vi "NMR T2 CPMG Sequence - Large Magnet - MC HPA (2W) - 2nd Setup.vi"() -> ()   [LabVIEW 2020]
uses:
  <instrlib>/niFgen/niFgen.llb/niFgen Output Mode.ctl
  <instrlib>/niFgen/niFgen.llb/niFgen Waveform Type.ctl
  <instrlib>/niFgen/niFgen.llb/niFgen_ctl Trigger DigEdge - Edge Values (Ring).ctl
  <instrlib>/niFgen/niFgen.llb/niFgen_ctl Trigger Source Values (Ring).ctl
  <instrlib>/niFgen/niFgen.llb/niFgen Trigger Mode.ctl
  <instrlib>/niScope/Controls/niScope acquisition type.ctl
  <instrlib>/niScope/Controls/niScope trigger slope.ctl
  <instrlib>/niScope/Controls/niScope trigger source.ctl
  <vilib>/Analysis/2dsp.llb/Integral Method.ctl
  <vilib>/Analysis/8numeric.llb/1D Numeric Integration.vi
  <vilib>/Utility/file.llb/Read Delimited Spreadsheet (DBL).vi
  <instrlib>/niFgen/niFgen.llb/niFgen Create Waveform (DBL).vi
  <instrlib>/niScope/Configure/Trigger/niScope Configure Trigger Edge.vi
  <instrlib>/niFgen/niFgen.llb/niFgen Configure Digital Edge Start Trigger.vi
  <instrlib>/niScope/Acquire/Fetch/niScope Fetch Cluster.vi
  <vilib>/Waveform/WDTFileIO.llb/Export Waveform To Spreadsheet File.vi
  <vilib>/Analysis/NI_AALPro.lvlib
panel:
  out "Pulse Echos - Current Scan":waveform(dbl)(graph)={"t0"=timestamp(0 s since 1904-01-01), "dt"=0.0012610340479192938, "Y"=array[3965 elements]} caption="Waveform Graph"
  in  "Write Output to File?":bool=TRUE
  out "Averaged T2 Decay":waveform(dbl)(graph)={"t0"=timestamp(0 s since 1904-01-01), "dt"=0.0012610340479192938, "Y"=array[3965 elements]} caption="Waveform Graph"
  out "Scan Number":i32=8
  out "Signal Intensity (Integral)":dbl=0.6544283602926818 format="%0.4f"
  out "Extracted T2 Decay - Current Scan":waveform(dbl)(graph)={"t0"=timestamp(0 s since 1904-01-01), "dt"=0.0012610340479192938, "Y"=array[3965 elements]} caption="Waveform Graph"
  in  "Pulse Train File":path=path "C:/Users/localuser/OneDrive - University of South Carolina/NMR Research/MATLAB/6 us 90 Degree - 1.25ms Tau - 3965 Pulses.txt"
  in  "Larmor Frequency":dbl=27410000.0 caption="Frequency" format="%.4p"
  in  "Number of Scans":i32=8
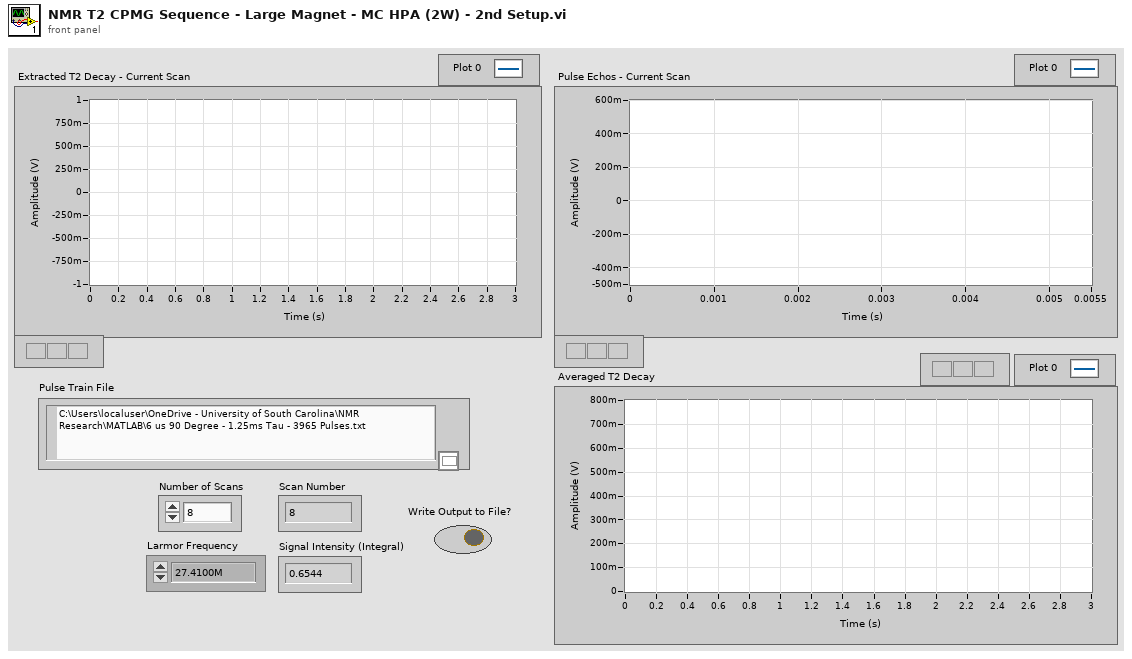
[diagram p1: front panel]
types:
  T1 = typedef "niFgen Output Mode.ctl" = u32
  T2 = typedef "niScope trigger source.ctl" = string
  T3 = typedef "niFgen_ctl Trigger Source Values (Ring).ctl" = string
  T4 = typedef "NI_AALPro.lvlib/Integral Method.ctl" = i32
  T5 = typedef "niScope trigger slope.ctl" = i32
  T6 = typedef "niScope acquisition type.ctl" = i32
  T7 = typedef "niFgen Trigger Mode.ctl" = i32
  T8 = typedef "niFgen_ctl Trigger DigEdge - Edge Values (Ring).ctl" = i32
  T9 = typedef "niFgen Waveform Type.ctl" = i32
  T10 = cluster{"relativeInitialX":dbl, "xIncrement":dbl, "wfm":dbl[]}
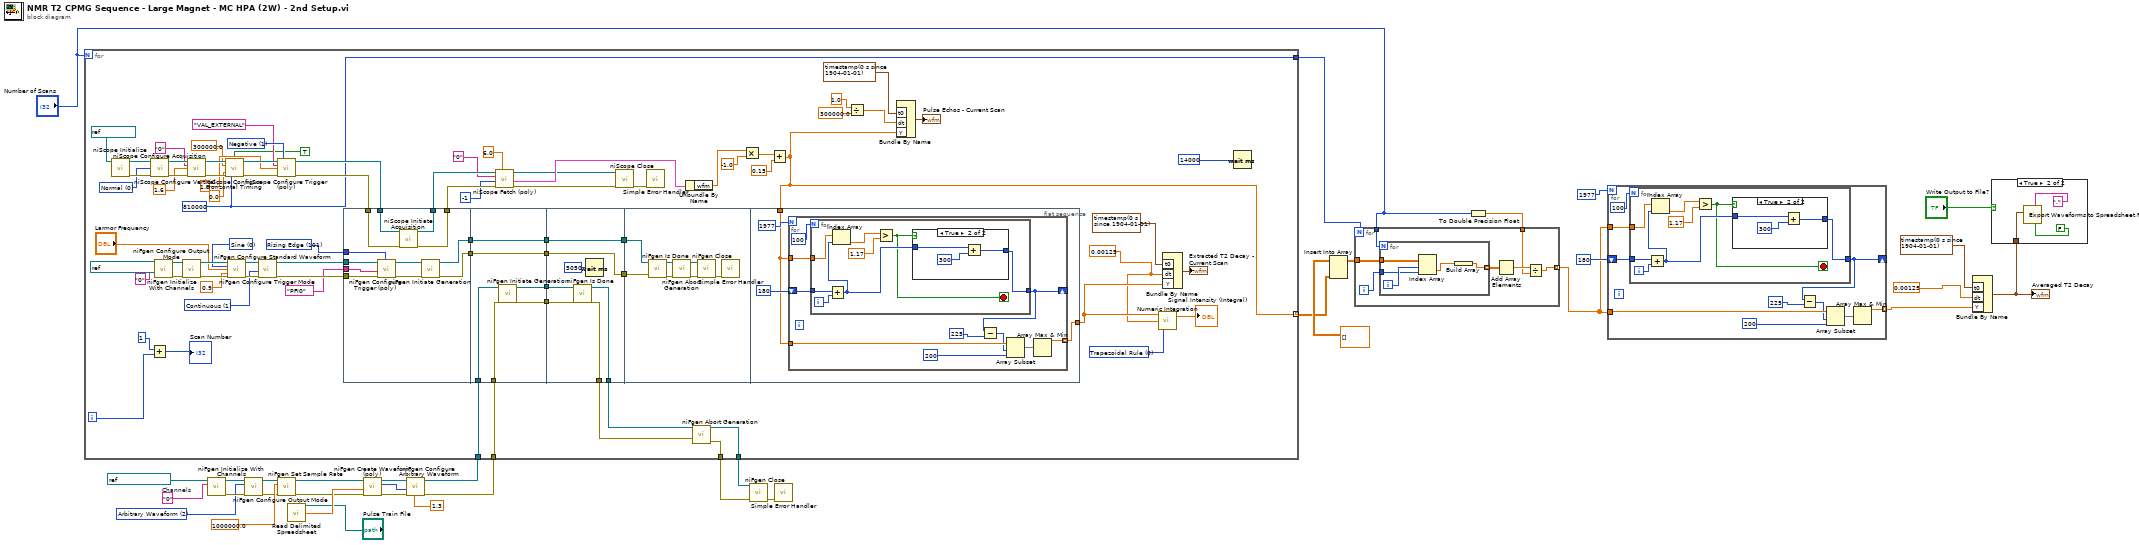
[diagram p0: block diagram]
diagram:
  w21 = "0"  # Channels
  w20 = T1 2 items=["Standard Function", "Frequency List", "Arbitrary Waveform", "Arbitrary Sequence", "Script"] ("output mode")
  n1 = call <instrlib>:"niFgen Initialize With Channels.vi"("Channel Name"=w21, "Resource Name"=refnum<k15> "PulseGenerator" ("FGEN Resource Name 2")) -> ("error out"=w24:errorcluster, "Instrument Handle Out"=w25:refnum<k15>)  [unwired: 8 in]
  n2 = call <instrlib>:"niFgen Configure Output Mode.vi"("error in (no error)"=w24, "Output Mode (default: 0=Standard Function)"=w20, "Instrument Handle"=w25) -> ("error out"=w28:errorcluster, "Instrument Handle Out"=w27:refnum<k15>)  [unwired: 6 in]
  n3 = call <instrlib>:"niFgen Set Sample Rate.vi"("error in (no error)"=w28, "Sample Rate (Samp/s)"=1000000.0 ("Sample Rate"), "Instrument Handle"=w27) -> ("error out"=w31:errorcluster, "Instrument Handle Out"=w30:refnum<k15>)  [unwired: 7 in]
  n4 = call-poly <vilib>:"Read Delimited Spreadsheet.vi"("file path (dialog if empty)"="Pulse Train File") -> ("first row"=w32:dbl[])  [unwired: 9 in, 5 out]
  n5 = call-poly <instrlib>:"niFgen Create Waveform (poly).vi"("error in (no error)"=w31, "Waveform Data Array"=w32, "Instrument Handle"=w30) -> ("error out"=w34:errorcluster, "Waveform Handle"=w35:i32, "Instrument Handle Out"=w33:refnum<k15>)  [unwired: 6 in]
  n6 = call <instrlib>:"niFgen Configure Arbitrary Waveform.vi"("Gain"=1.3, "error in (no error)"=w34, "Waveform Handle"=w35, "Instrument Handle"=w33) -> ("error out"=w19:errorcluster, "Instrument Handle Out"=w18:refnum<k15>)  [unwired: 6 in]
  n7 = for {
    N: "Number of Scans" -> [_]
    tunnel: w19 -> [w97]
    tunnel: w18 -> [w96]
    tunnel: [w95] -> w16
    tunnel: [w94] -> w15
    tunnel: [w37] -> w12 mode=indexing
    tunnel: [w48] -> w9
    i -> [w55]
    w57 = T4 0 items=["Trapezoidal Rule", "Simpson's Rule", "Simpson's 3/8 Rule", "Bode Rule"] ("integration method")
    w36 = 0.00125 ("y")
    w48 = 810000 ("min record length")
    w82 = T5 1 items=["Positive", "Negative"] ("trigger slope")
    w83 = T6 0 items=["Normal"=0, "Flex Res"=1, "DDC"=3] ("acquisition Type")
    w102 = T7 1 items=["Single", "Continuous", "Stepped", "Burst"] ("Trigger Mode (default: 1=continuous)")
    w106 = T8 101 items=["Rising Edge"=101, "Falling Edge"=102] ("Edge (Rising)")
    w107 = T9 0 items=["Sine", "Square", "Triangle", "Ramp Up", "Ramp Down", "DC", "Noise", "User"] ("Waveform")
    n8 = call <instrlib>:"niScope Initialize.vi"("resource name"=refnum<k15> "PXI1Slot6") -> ("instrument handle"=w84:refnum<k15>, "error out"=w85:errorcluster)  [unwired: 13 in]
    n9 = call <instrlib>:"niScope Configure Acquisition.vi"("instrument handle"=w84, "acquisition Type"=w83, "error in"=w85) -> ("instrument handle out"=w87:refnum<k15>, "error out"=w88:errorcluster)  [unwired: 11 in]
    n10 = Add(x=1, y=w55) -> (x+y=→"Scan Number":i32)
    n11 = call <instrlib>:"niFgen Initialize With Channels.vi"("Channel Name"="0", "Resource Name"=refnum<k15> "SinWaveGenerator" ("Sine Wave Module")) -> ("error out"=w112:errorcluster, "Instrument Handle Out"=w115:refnum<k15>)  [unwired: 8 in]
    n12 = call <instrlib>:"niFgen Configure Output Mode.vi"("error in (no error)"=w112, "Instrument Handle"=w115) -> ("error out"=w111:errorcluster, "Instrument Handle Out"=w114:refnum<k15>)  [unwired: 7 in]
    n13 = call <instrlib>:"niScope Configure Vertical.vi"("instrument handle"=w87, "channels"="0", "vertical range"=1.6, "error in"=w88) -> ("instrument handle out"=w89:refnum<k15>, "error out"=w90:errorcluster)  [unwired: 10 in]
    n14 = call <instrlib>:"niScope Configure Horizontal Timing.vi"("instrument handle"=w89, "enforce realtime"=TRUE, "min sample rate"=300000.0, "reference position"=0.0, "error in"=w90, "min record length"=w48) -> ("instrument handle out"=w91:refnum<k15>, "error out"=w92:errorcluster)  [unwired: 8 in]
    n15 = call <instrlib>:"niFgen Configure Standard Waveform.vi"("Instrument Handle"=w114, "Waveform"=w107, "Frequency"="Larmor Frequency", "Amplitude"=0.9, "error in (no error)"=w111) -> ("Instrument Handle Out"=w113:refnum<k15>, "error out"=w110:errorcluster)  [unwired: 9 in]
    n16 = call <instrlib>:"niFgen Configure Trigger Mode.vi"("error in (no error)"=w110, "Trigger Mode (default: 1=continuous)"=w102, "Instrument Handle"=w113) -> ("error out"=w105:errorcluster, "Instrument Handle Out"=w103:refnum<k15>)  [unwired: 7 in]
    n17 = call-poly <instrlib>:"niScope Configure Trigger (poly).vi"("instrument handle"=w91, "trigger slope"=w82, "trigger source"=T2 "VAL_EXTERNAL", "trigger level"=1.0, "error in"=w92) -> ("instrument handle out"=w76:refnum<k15>, "error out"=w75:errorcluster)  [unwired: 9 in]
    n18 = flat-sequence {
      tunnel: w106 -> [w126]
      tunnel: w105 -> [w125]
      tunnel: T3 "PFI0" ("Source") -> [w124]
      tunnel: w103 -> [w123]
      tunnel: w76 -> [w121]
      tunnel: w75 -> [w120]
      tunnel: [w119] -> w74
      tunnel: [w118] -> w73
      tunnel: [w117] -> w63
      tunnel: [w116] -> w60
      tunnel: w97 -> [w133]
      tunnel: w96 -> [w132]
      tunnel: [w131] -> w67
      tunnel: [w130] -> w66
      tunnel: [w129] -> w64
      tunnel: w63 -> [w129]
      tunnel: [w128] -> w61
      tunnel: w60 -> [w128]
      tunnel: [w139] -> w100
      tunnel: [w138] -> w99
      tunnel: w67 -> [w137]
      tunnel: w66 -> [w136]
      tunnel: [w135] -> w65
      tunnel: w64 -> [w135]
      tunnel: [w134] -> w62
      tunnel: w61 -> [w134]
      tunnel: w65 -> [w142]
      tunnel: w62 -> [w141]
      tunnel: w37 -> [w148]
      tunnel: [w150] -> w47
      frame #0 {
        n19 = call-poly <instrlib>:"niFgen Configure Trigger (poly).vi"("Edge (Rising)"=w126, "error in (no error)"=w125, "Source"=w124, "Instrument Handle"=w123) -> ("error out"=w122:errorcluster, "Instrument Handle Out"=w127:refnum<k15>)  [unwired: 6 in]
        n20 = call <instrlib>:"niScope Initiate Acquisition.vi"("instrument handle"=w121, "error in"=w120) -> ("instrument handle out"=w119:refnum<k15>, "error out"=w118:errorcluster)  [unwired: 12 in]
        n21 = call <instrlib>:"niFgen Initiate Generation.vi"("error in (no error)"=w122, "Instrument Handle"=w127) -> ("error out"=w116:errorcluster, "Instrument Handle Out"=w117:refnum<k15>)  [unwired: 8 in]
      }
      frame #1 {
        n22 = call <instrlib>:"niFgen Initiate Generation.vi"("error in (no error)"=w133, "Instrument Handle"=w132) -> ("error out"=w130:errorcluster, "Instrument Handle Out"=w131:refnum<k15>)  [unwired: 8 in]
      }
      frame #2 {
        n23 = call <instrlib>:"niFgen Is Done.vi"("error in (no error)"=w136, "Instrument Handle"=w137) -> ("error out"=w139:errorcluster, "Instrument Handle Out"=w138:refnum<k15>)  [unwired: 7 in, 1 out]
        n24 = Wait (ms)(milliseconds to wait=u32 5050) -> ()  [unwired: 1 out]
      }
      frame #3 {
        n25 = call <instrlib>:"niFgen Is Done.vi"("error in (no error)"=w141, "Instrument Handle"=w142) -> ("error out"=w145:errorcluster, "Instrument Handle Out"=w144:refnum<k15>)  [unwired: 7 in, 1 out]
        n26 = call <instrlib>:"niFgen Abort Generation.vi"("error in (no error)"=w145, "Instrument Handle"=w144) -> ("error out"=w146:errorcluster, "Instrument Handle Out"=w147:refnum<k15>)  [unwired: 8 in]
        n27 = call <instrlib>:"niFgen Close.vi"("error in (no error)"=w146, "Instrument Handle"=w147) -> ("error out"=w143:errorcluster)  [unwired: 9 in]
        n28 = call <vilib>:"Simple Error Handler.vi"("error in (no error)"=w143) -> ()  [unwired: 4 in, 5 out]
      }
      frame #4 {
        n29 = for {
          N: 1977 -> [_]
          tunnel: [w160] -> w150 mode=indexing
          tunnel: w148 -> [w159]
          shift-right: [w154] -> _
          shift-left: 180 -> [w155]
          tunnel: w148 -> [w153]
          n30 = for {
            N: 100 -> [_]
            tunnel: w153 -> [w165]
            tunnel: w155 -> [w168]
            tunnel: [w163] -> w154
            i -> [w169]
            stop <- w162 stop-if-true
            n31 = Add(x=w168, y=w169) -> (x+y=w164:i32)
            n32 = Index Array(array=w165, index=w164) -> (element=w166:dbl)
            n33 = Greater?(x=w166, y=1.17) -> (0:w162:bool)
            n34 = case shown="True" w162 {
              tunnel: w164 -> [w170 w171]
              tunnel: [w170 w173] -> w163
              frame False {
              }
              frame True {
                n35 = Add(x=w171, y=300) -> (x+y=w173:i32)
              }
            }
          }
          n36 = Subtract(x=w154, y=225) -> (x-y=w156:i32)
          n37 = Array Subset(array=w159, index=w156, length=200 ("y")) -> (w161:dbl[])
          n38 = Array Max & Min(array=w161) -> (max value=w160:dbl)  [unwired: 3 out]
        }
      }
    }
    n39 = call-poly <instrlib>:"niScope Fetch (poly).vi"("timeout"=6.0, "error in"=w73, "numSamples"=-1, "channels"="0", "instrument handle"=w74) -> ("error out"=w49:errorcluster, "waveform"=w52:T10, "instrument handle out"=w50:refnum<k15>)  [unwired: 3 in, 1 out]
    n40 = call <instrlib>:"niScope Close.vi"("instrument handle"=w50, "error in"=w49) -> ("error out"=w93:errorcluster)  [unwired: 13 in]
    n41 = call <vilib>:"Simple Error Handler.vi"("error in (no error)"=w93) -> ()  [unwired: 4 in, 5 out]
    n42 = Unbundle By Name(w52) -> ("wfm"=w41:dbl[])
    n43 = call <instrlib>:"niFgen Abort Generation.vi"("error in (no error)"=w100, "Instrument Handle"=w99) -> ("error out"=w95:errorcluster, "Instrument Handle Out"=w94:refnum<k15>)  [unwired: 8 in]
    n44 = Multiply(x=w41, y=-1.0) -> (x*y=w38:dbl[])
    n45 = Add(x=w38, y=0.15) -> (x+y=w37:dbl[])
    n46 = Divide(x=1.0, y=300000.0) -> (x/y=w42:dbl)
    n47 = Bundle By Name("t0"=timestamp(0 s since 1904-01-01), "dt"=w42, "Y"=w37) -> (→"Pulse Echos - Current Scan":waveform(dbl))  [unwired: 1 in]
    n48 = call-poly <vilib>:"Numeric Integration.vi"("integration method"=w57, "dt"=w36, "Input Array"=w47) -> ("result"=→"Signal Intensity (Integral)":dbl)  [unwired: 1 out]
    n49 = Bundle By Name("t0"=timestamp(0 s since 1904-01-01), "dt"=w36, "Y"=w47) -> (→"Extracted T2 Decay - Current Scan":waveform(dbl))  [unwired: 1 in]
    n50 = Wait (ms)(milliseconds to wait=u32 14000 ("Delay Time (ms)")) -> ()  [unwired: 1 out]
  }
  n51 = call <instrlib>:"niFgen Close.vi"("error in (no error)"=w16, "Instrument Handle"=w15) -> ("error out"=w17:errorcluster)  [unwired: 9 in]
  n52 = call <vilib>:"Simple Error Handler.vi"("error in (no error)"=w17) -> ()  [unwired: 4 in, 5 out]
  n53 = Insert Into Array(array=dbl[][] [], new element=w12) -> (w14:dbl[][])  [unwired: 2 in]
  n54 = To Double Precision Float(number="Number of Scans") -> (double precision float=w11:dbl)
  n55 = for {
    N: w9 -> [_]
    tunnel: w14 -> [w180]
    tunnel: [w176] -> w5 mode=indexing
    tunnel: "Number of Scans" -> [w175]
    tunnel: w11 -> [w174]
    i -> [w179]
    n56 = for {
      N: w175 -> [_]
      tunnel: w180 -> [w185]
      tunnel: w179 -> [w183]
      tunnel: [w181] -> w178 mode=indexing
      i -> [w184]
      n57 = Index Array(array=w185, index (row)=w184, index (col)=w183) -> (element=w182:dbl)
      n58 = Build Array(w182) -> (w181:dbl[])
    }
    n59 = Add Array Elements(numeric array=w178) -> (sum=w177:dbl)
    n60 = Divide(x=w177, y=w174) -> (x/y=w176:dbl)
  }
  n61 = for {
    N: 1977 -> [_]
    tunnel: [w194] -> w4 mode=indexing
    tunnel: w5 -> [w193]
    shift-right: [w188] -> _
    shift-left: 180 -> [w189]
    tunnel: w5 -> [w187]
    n62 = for {
      N: 100 -> [_]
      tunnel: w187 -> [w199]
      tunnel: w189 -> [w202]
      tunnel: [w197] -> w188
      i -> [w203]
      stop <- w196 stop-if-true
      n63 = Add(x=w202, y=w203) -> (x+y=w198:i32)
      n64 = Index Array(array=w199, index=w198) -> (element=w200:dbl)
      n65 = Greater?(x=w200, y=1.17) -> (0:w196:bool)
      n66 = case shown="True" w196 {
        tunnel: w198 -> [w204 w205]
        tunnel: [w204 w207] -> w197
        frame False {
        }
        frame True {
          n67 = Add(x=w205, y=300) -> (x+y=w207:i32)
        }
      }
    }
    n68 = Subtract(x=w188, y=225) -> (x-y=w190:i32)
    n69 = Array Subset(array=w193, index=w190, length=200 ("y")) -> (w195:dbl[])
    n70 = Array Max & Min(array=w195) -> (max value=w194:dbl)  [unwired: 3 out]
  }
  n71 = Bundle By Name("t0"=timestamp(0 s since 1904-01-01), "dt"=0.00125 ("y"), "Y"=w4) -> (w2:waveform(dbl))  [unwired: 1 in]
  "Averaged T2 Decay" <- w2
  n72 = case shown="True" "Write Output to File?" {
    tunnel: w2 -> [_ w208]
    frame False {
    }
    frame True {
      n73 = call-poly <vilib>:"Export Waveforms to Spreadsheet File.vi"("header? (write header:T)"=FALSE, "delimiter (Tab)"=",", "waveform"=w208) -> ()  [unwired: 7 in, 2 out]
    }
  }
